vi "Create Instance.vi"(8 "error in (no error)":errorcluster) -> (0 "error out":errorcluster, 3 "PrefsDB out":refnum<class "PrefsDB.lvclass">)   [LabVIEW 2020, in "User Prefs.lvlib" / "PrefsDB.lvclass"]
uses:
  PrefsDB.lvclass
  PrefsDB.lvclass/PrefsDB.ctl
  lv-cdm/CDM-Config/Config Manager/Config Manager.lvclass
  Ref Data.ctl
  Pref Group.ctl
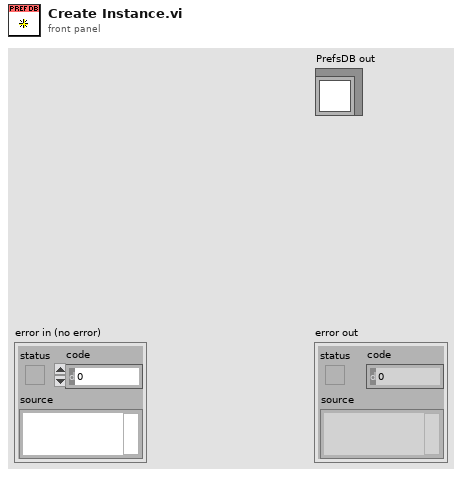
[diagram p1: front panel]
types:
  T1 = typedef "User Prefs.lvlib/PrefsDB.lvclass/Ref Data.ctl" = cluster{"Map":map{string, T2}}
  T2 = typedef "User Prefs.lvlib/PrefsDB.lvclass/Pref Group.ctl" = cluster{"Config Manager":refnum<class "Config Manager.lvclass">, "Group":string}
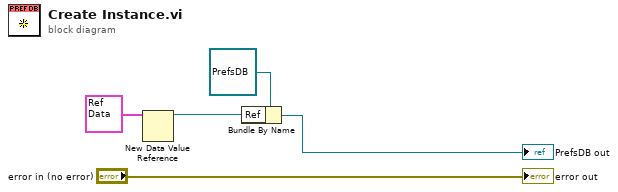
[diagram p0: block diagram]
diagram:
  n1 = New Data Value Reference(data value=T1 {"Map"={}} ("Ref Data")) -> (data value reference=w1:refnum<data-value>)  [unwired: 1 in, 1 out]
  n2 = Bundle By Name(cluster=refnum<class "PrefsDB.lvclass"> refnum ("PrefsDB in"), "Ref"=w1) -> (→"PrefsDB out":refnum<class "PrefsDB.lvclass">)
  "error out" <- "error in (no error)"
